vi "Property Tree_Select on Enter.vi"(7 "Save Action":T1=enum."Wire Unbundle", 11 "Tree Ref":refnum<vi>[](array[refnum])) -> ()   [LabVIEW 2023]
doc: "When enter button is pressed, check for selected item and add to selected properties if unchecked. Use R or W if only one or the other posible, and present dialog if both are possible."
uses:
  controls/action enum.ctl
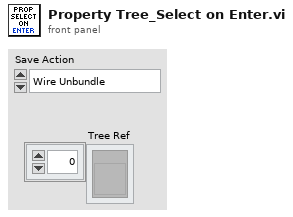
[diagram p1: front panel]
types:
  T1 = typedef "action enum.ctl" = enum16{"[NONE]", "Wire Bundle", "Wire Unbundle", "Terminal Unbundle", "Terminal Bundle", "Bundler Move Up", "Bundler Move Down", "Bundler Insert", "Bundler Remove", "Bundler Remove Unwired", "Bundler Rearrange", "In Place Insert", "In Place Remove", "In Place Remove Unwired", "In Place Rearrange", "Wire Properties", "Wire Method", "Terminal Properties", "Terminal Method", "Property Move Up", "Property Move Down", "Properties Insert", "Properties Remove", "Properties Remove Unwired", "Properties Rearrange", "Method Change", "Class for Constant", "Class For Control", "Class For Node", "Class Name to Clipboard"}
  T2 = cluster{"Can R":bool, "Can W":bool, "Is R":bool, "Is W":bool}
  T3 = enum16{"Init", "Read", "Remove", "Remove or Append", "Append", "Append If New"}
  T4 = enum16{"Left Button", "Center Button", "Right Button", "Window Close"}
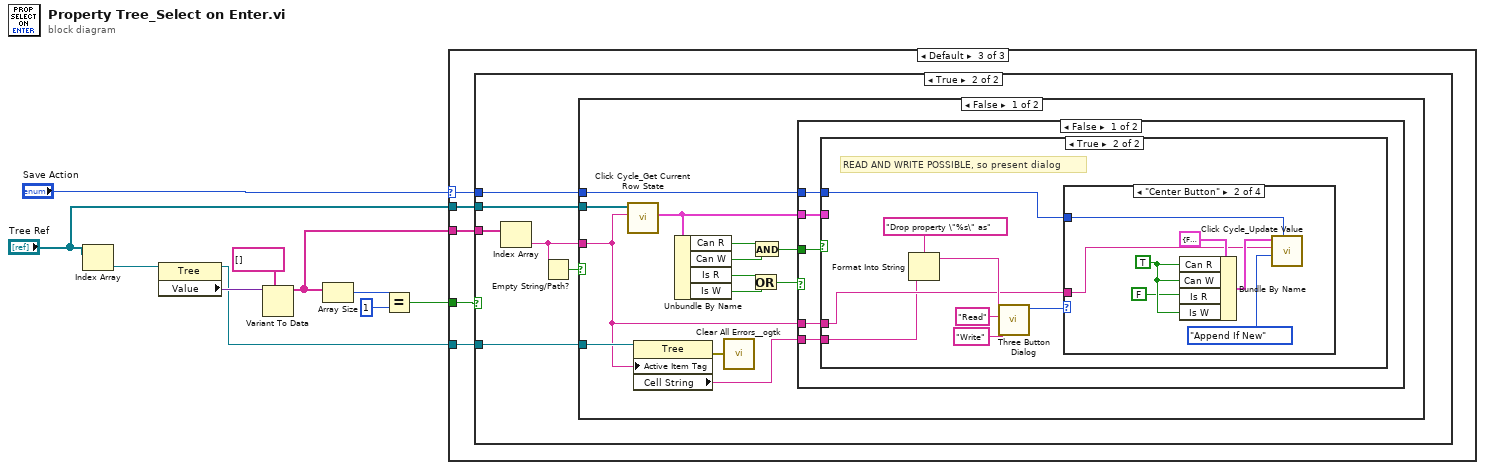
[diagram p0: block diagram]
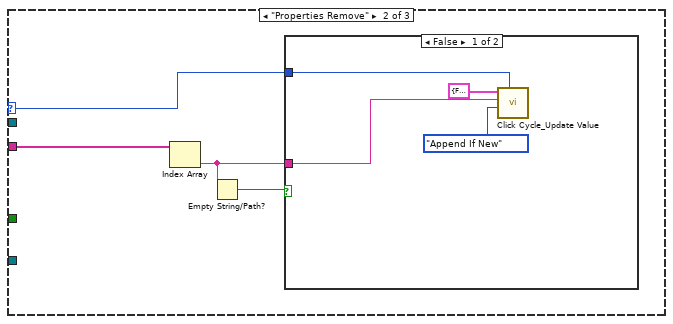
[diagram p3: hidden frame]
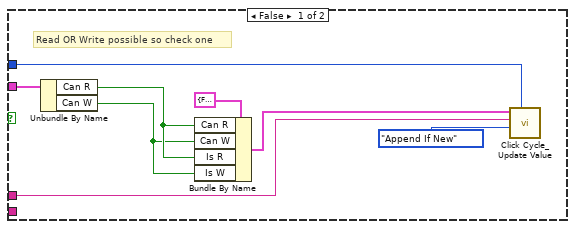
[diagram p6: hidden frame]
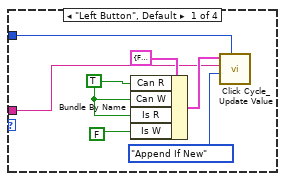
[diagram p7: hidden frame]
diagram:
  n1 = Index Array(array="Tree Ref") -> (element=w10:refnum<vi>)  [unwired: 1 in]
  n2 = property class="Tree"(reference=w10) -> (reference out=w2:refnum<vi>, "Value"=w9:variant)  [unwired: 1 in, 1 out]
  n3 = Variant To Data(type=string[] [], Variant=w9) -> (data=w3:string[])  [unwired: 1 in, 1 out]
  n4 = Array Size(array=w3) -> (size(s)=w7:i32)
  n5 = Equal?(x=w7, y=1) -> (x = y?=w4:bool)
  n6 = case shown="Default" "Save Action" {
    selector: "Save Action" -> [_ w11 w19]
    tunnel: "Tree Ref" -> [_ _ w23]
    tunnel: w4 -> [_ _ w22]
    tunnel: w3 -> [_ w14 w21]
    tunnel: w2 -> [_ _ w20]
    frame "Properties Rearrange" {
    }
    frame "Properties Remove" {
      n7 = Index Array(array=w14) -> (element=w12:string)  [unwired: 1 in]
      n8 = Empty String/Path?(string/path=w12) -> (empty?=w13:bool)
      n9 = case shown="False" w13 {
        tunnel: w12 -> [w17 _]
        tunnel: w11 -> [w15 _]
        frame False {
          n10 = call "Click Cycle_Update Value.vi"("Action"=w15, "Save Action"=T3."Append If New" ("Action"), "Tag"=w17, "Row RW State"=T2 {"Can R"=FALSE, "Can W"=FALSE, "Is R"=FALSE, "Is W"=FALSE}) -> ()  [unwired: 7 in, 1 out]
        }
        frame True {
        }
      }
    }
    frame Default {
      n11 = case shown="True" w22 {
        tunnel: w23 -> [_ w29]
        tunnel: w21 -> [_ w28]
        tunnel: w20 -> [_ w27]
        tunnel: w19 -> [_ w24]
        frame False {
        }
        frame True {
          n12 = Index Array(array=w28) -> (element=w26:string)  [unwired: 1 in]
          n13 = Empty String/Path?(string/path=w26) -> (empty?=w25:bool)
          n14 = case shown="False" w25 {
            tunnel: w29 -> [w42 _]
            tunnel: w27 -> [w34 _]
            tunnel: w26 -> [w33 _]
            tunnel: w24 -> [w30 _]
            frame False {
              n15 = call "Click Cycle_Get Current Row State.vi"("Active Item:Tag"=w33, "All Tree Refs"=w42) -> ("Row RW State"=w35:T2)  [unwired: 7 in, 2 out]
              n16 = property class="Tree"(reference=w34, "Active Item Tag"=w33) -> (error out=w31:errorcluster, "Cell String"=w32:string)  [unwired: 1 in, 1 out]
              n17 = Unbundle By Name(w35) -> ("Can R"=w39:bool, "Can W"=w38:bool, "Is R"=w41:bool, "Is W"=w40:bool)
              n18 = call <userlib>:"Clear All Errors__ogtk.vi"("Error In"=w31) -> ()  [unwired: 3 in, 1 out]
              n19 = Or(x=w41, y=w40) -> (x .or. y?=w37:bool)
              n20 = And(x=w39, y=w38) -> (x .and. y?=w36:bool)
              n21 = case shown="False" w37 {
                tunnel: w36 -> [w47 _]
                tunnel: w35 -> [w46 _]
                tunnel: w33 -> [w45 _]
                tunnel: w32 -> [w44 _]
                tunnel: w30 -> [w43 _]
                frame False {
                  n22 = case shown="True" w47 {
                    tunnel: w46 -> [w55 _]
                    tunnel: w45 -> [w50 w58]
                    tunnel: w44 -> [_ w57]
                    tunnel: w43 -> [w48 w56]
                    frame False {
                      # "Read OR Write possible so check one"
                      n23 = Unbundle By Name(w55) -> ("Can R"=w52:bool, "Can W"=w51:bool)
                      n24 = Bundle By Name(cluster=T2 {"Can R"=FALSE, "Can W"=FALSE, "Is R"=FALSE, "Is W"=FALSE} ("Row RW State"), "Can R"=w52, "Can W"=w51, "Is R"=w52, "Is W"=w51) -> (w54:T2)
                      n25 = call "Click Cycle_Update Value.vi"("Action"=w48, "Save Action"=T3."Append If New" ("Action"), "Tag"=w50, "Row RW State"=w54) -> ()  [unwired: 7 in, 1 out]
                    }
                    frame True {
                      # "READ AND WRITE POSSIBLE, so present dialog"
                      n26 = Format Into String(format string="Drop property \"%s\" as", w57) -> (resulting string=w60:string)  [unwired: 2 in, 1 out]
                      n27 = call <vilib>:"Three Button Dialog.vi"("Center Button Text (\"No\")"="Write" ("Center Button Text (\"No\")"), "Left Button Text (\"Yes\")"="Read" ("Left Button Text (\"Yes\")"), "message"=w60) -> ("Which Button?"=w59:T4)  [unwired: 8 in]
                      n28 = case shown="\"Center Button\"" w59 {
                        tunnel: w58 -> [w66 w75 _ _]
                        tunnel: w56 -> [w64 w71 _ _]
                        frame "Left Button", Default {
                          w68 = TRUE
                          n29 = Bundle By Name(cluster=T2 {"Can R"=FALSE, "Can W"=FALSE, "Is R"=FALSE, "Is W"=FALSE} ("Row RW State"), "Can R"=w68, "Can W"=w68, "Is R"=w68, "Is W"=FALSE) -> (w70:T2)
                          n30 = call "Click Cycle_Update Value.vi"("Action"=w64, "Save Action"=T3."Append If New" ("Action"), "Tag"=w66, "Row RW State"=w70) -> ()  [unwired: 7 in, 1 out]
                        }
                        frame "Center Button" {
                          w74 = TRUE
                          n31 = Bundle By Name(cluster=T2 {"Can R"=FALSE, "Can W"=FALSE, "Is R"=FALSE, "Is W"=FALSE} ("Row RW State"), "Can R"=w74, "Can W"=w74, "Is R"=FALSE, "Is W"=w74) -> (w77:T2)
                          n32 = call "Click Cycle_Update Value.vi"("Action"=w71, "Save Action"=T3."Append If New" ("Action"), "Tag"=w75, "Row RW State"=w77) -> ()  [unwired: 7 in, 1 out]
                        }
                        frame "Right Button" {
                        }
                        frame "Window Close" {
                        }
                      }
                    }
                  }
                }
                frame True {
                  # "Already selected, do nothing"
                }
              }
            }
            frame True {
            }
          }
        }
      }
    }
  }
